vi "ImPro - Init UI.vi"(8 "error in (no error)":errorcluster, 11 "UI Refs":T2) -> (0 "error out":errorcluster, 1 "All Filenames":string[](array[string]), 2 "Image index":i32, 3 "ImProSettings Out":T1)   [LabVIEW 2023]
uses:
  Controls/ImPro - UI Refs.ctl
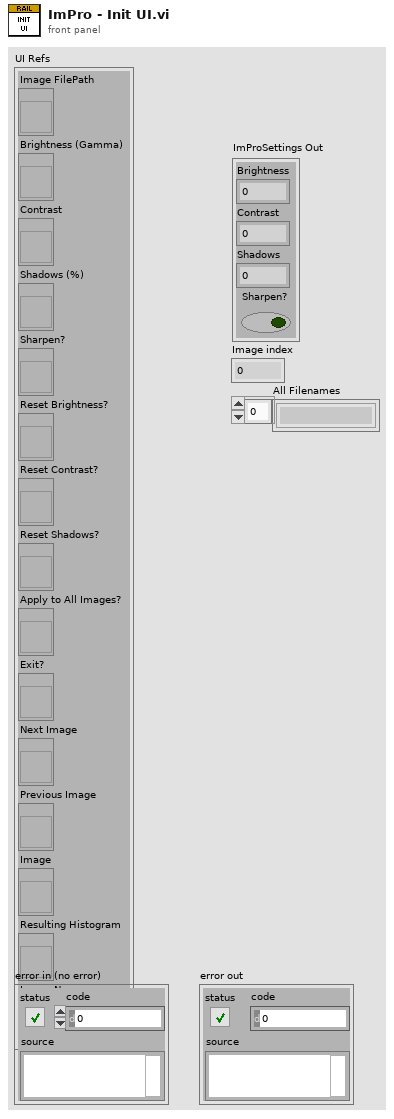
[diagram p1: front panel]
types:
  T1 = cluster{"Brightness":dbl, "Contrast":dbl, "Shadows":dbl, "Sharpen?":bool}
  T2 = typedef "ImPro - UI Refs.ctl" = cluster{"Image FilePath":refnum<vi>, "Brightness (Gamma)":refnum<vi>, "Contrast":refnum<vi>, "Shadows (%)":refnum<vi>, "Sharpen?":refnum<vi>, "Reset Brightness?":refnum<vi>, "Reset Contrast?":refnum<vi>, "Reset Shadows?":refnum<vi>, "Apply to All Images?":refnum<vi>, "Exit?":refnum<vi>, "Next Image":refnum<vi>, "Previous Image":refnum<vi>, "Image":refnum<vi>, "Resulting Histogram":refnum<vi>, "Image Name":refnum<vi>}
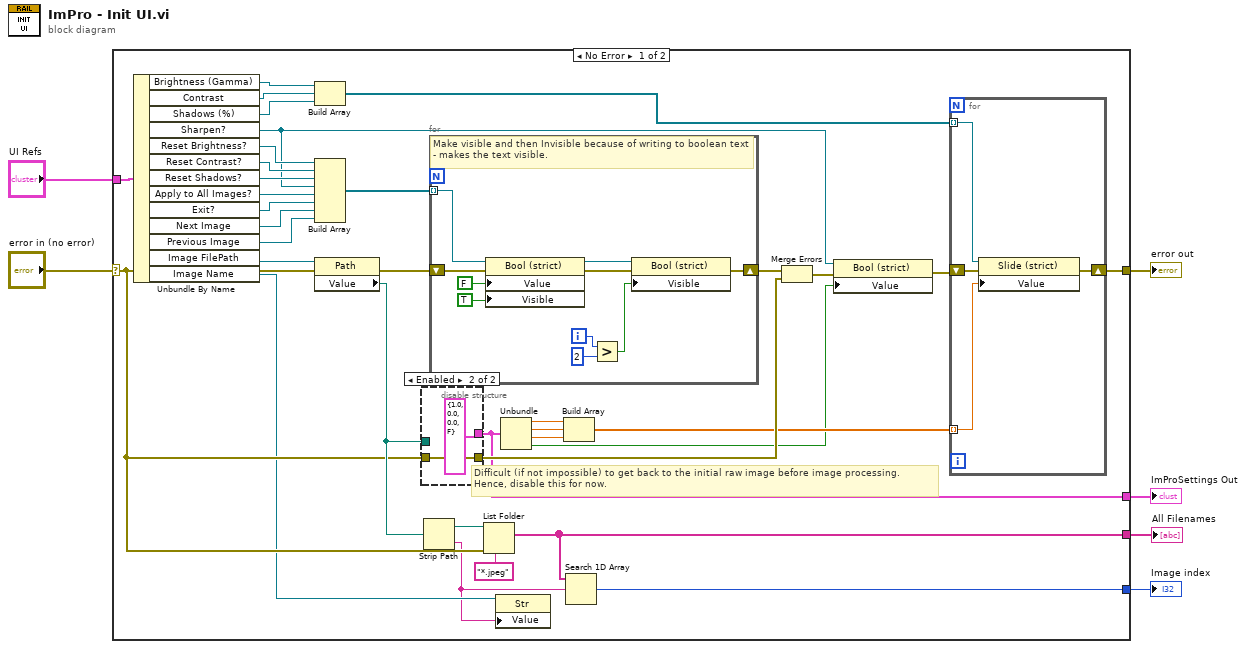
[diagram p0: block diagram]
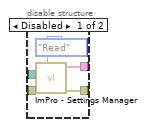
[diagram p2: hidden frame]
diagram:
  n1 = case shown="No Error" "error in (no error)" {
    selector: "error in (no error)" -> [w12 w63]
    tunnel: [w29 w63] -> w5
    tunnel: "UI Refs" -> [w41 _]
    tunnel: [w17 _] -> w3
    tunnel: [w8 _] -> w2
    tunnel: [w7 _] -> w1
    frame No Error {
      # "Difficult (if not impossible) to get back to the initial raw image before image processing.\nHence, disable this for now."
      n2 = Unbundle By Name(w41) -> ("Brightness (Gamma)"=w32:refnum<vi>, "Contrast"=w33:refnum<vi>, "Shadows (%)"=w34:refnum<vi>, "Sharpen?"=w19:refnum<vi>, "Reset Brightness?"=w40:refnum<vi>, "Reset Contrast?"=w39:refnum<vi>, "Reset Shadows?"=w38:refnum<vi>, "Apply to All Images?"=w37:refnum<vi>, "Exit?"=w36:refnum<vi>, "Next Image"=w16:refnum<vi>, "Previous Image"=w15:refnum<vi>, "Image FilePath"=w28:refnum<vi>, "Image Name"=w10:refnum<vi>)
      n3 = Build Array(w32, w33, w34) -> (w30:refnum<vi>[])
      n4 = Build Array(w40, w39, w38, w19, w37, w36, w16, w15) -> (w35:refnum<vi>[])
      n5 = property class="Path"(reference=w28, error in=w12) -> (error out=w27:errorcluster, "Value"=w14:path)  [unwired: 1 out]
      n6 = disable-structure shown="Enabled" {
        disable-tunnel: w12 -> [w46 w48]
        disable-tunnel: w14 -> [w45 _]
        disable-tunnel: [w43 w48] -> w26
        disable-tunnel: [w42 T1 {"Brightness"=1.0, "Contrast"=0.0, "Shadows"=0.0, "Sharpen?"=FALSE} ("ImProSettings Out")] -> w17
        frame Disabled {
          n7 = call "ImPro - Settings Manager.vi"("Command"=enum16{"Read", "Write"}."Read", "error in (no error)"=w46, "ImagePath"=w45) -> ("error out"=w43:errorcluster, "ImProSettings Out"=w42:T1)  [unwired: 7 in]
        }
        frame Enabled {
        }
      }
      n8 = Strip Path(path=w14) -> (stripped path=w13:path, name=w9:string)
      n9 = for {
        tunnel: w35 -> [w58] mode=indexing
        shift-right: [w52] -> w31
        shift-left: w27 -> [w56]
        i -> [w55]
        # "Make visible and then Invisible because of writing to boolean text - makes the text visible."
        n10 = property class="Bool (strict)"(reference=w58, error in=w56, "Value"=FALSE, "Visible"=TRUE) -> (reference out=w49:refnum<vi>, error out=w53:errorcluster)
        n11 = Greater?(x=w55, y=2) -> (0:w51:bool)
        n12 = property class="Bool (strict)"(reference=w49, error in=w53, "Visible"=w51) -> (error out=w52:errorcluster)  [unwired: 1 out]
      }
      n13 = List Folder(path=w13, pattern="*.jpeg", error in=w12) -> (filenames=w7:string[])  [unwired: 1 in, 3 out]
      n14 = property class="Str"(reference=w10, "Value"=w9) -> ()  [unwired: 1 in, 2 out]
      n15 = Unbundle(w17) -> ("Brightness"=w25:dbl, "Contrast"=w22:dbl, "Shadows"=w23:dbl, "Sharpen?"=w18:bool)
      n16 = Build Array(w25, w22, w23) -> (w24:dbl[])
      n17 = Search 1D Array(1D array=w7, element=w9) -> (index of element=w8:i32)  [unwired: 1 in]
      n18 = Merge Errors(w31, w26) -> (w21:errorcluster)
      n19 = property class="Bool (strict)"(reference=w19, error in=w21, "Value"=w18) -> (error out=w20:errorcluster)  [unwired: 1 out]
      n20 = for {
        tunnel: w30 -> [w62] mode=indexing
        shift-right: [w60] -> w29
        shift-left: w20 -> [w61]
        tunnel: w24 -> [w59] mode=indexing
        n21 = property class="Slide (strict)"(reference=w62, error in=w61, "Value"=w59) -> (error out=w60:errorcluster)  [unwired: 1 out]
      }
    }
    frame Error {
    }
  }
  "error out" <- w5
  "ImProSettings Out" <- w3
  "Image index" <- w2
  "All Filenames" <- w1
